vi "SUB_COM_ESC1_NEW.vi"(3 "duplicate VISA resource name":refnum<visa-resource-name>) -> (0 "OUT string":string, 1 "VISA resource OUT":refnum<visa-resource-name>)   [LabVIEW 2011]
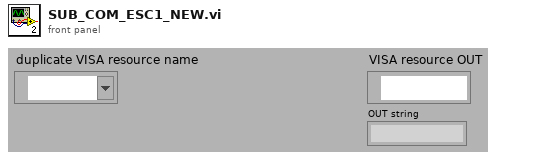
[diagram p1: front panel]
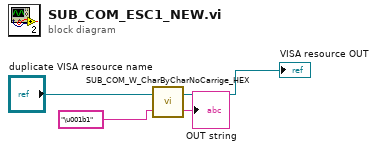
[diagram p0: block diagram]
diagram:
  n1 = call "SUB_COM_W_CharByCharNoCarrige_HEX.vi"("cmd string"="\u001b1" ("write buffer"), "duplicate VISA resource name"="duplicate VISA resource name") -> ("OUT string"=→"OUT string":string, "VISA resource OUT"=→"VISA resource OUT":refnum<visa-resource-name>)
